vi "ObtainPrivateQueues.vi"(8 "error in (no error)":errorcluster, 11 "DAQmx":refnum<class "DAQmx.lvclass">) -> (0 "error out":errorcluster, 3 "DAQmx out":refnum<class "DAQmx.lvclass">)   [LabVIEW 2019, in "DAQmx.lvclass"]
uses:
  DAQmx.lvclass
  typedefs/DAQmx.States--enum.ctl
  typedefs/DAQ.Config.AO--Cluster--Array.ctl
  typedefs/DAQ.Config.AO--Cluster.ctl
  typedefs/DAQ.Config.AO.Range--enum.ctl
  typedefs/DAQ.Config.Device Type--enum.ctl
  typedefs/DAQ.Config.AI--Cluster--Array.ctl
  typedefs/DAQ.Config.AI--Cluster.ctl
  typedefs/DAQ.Config.AI.Coupling--enum.ctl
  typedefs/DAQ.Config.AI.Range--enum.ctl
  typedefs/DAQ.Config.Timing--Cluster.ctl
  typedefs/DAQ.Config.Timing.Sampling--Cluster.ctl
  typedefs/DAQ.Config.Timing.Fs Mode--enum.ctl
  DAQmx.lvclass/DAQmx.ctl
panel:
  # "For instructions on how to use the JKI State Machine Objects, examples and video tutorials, visit:\nhttp://jki.net/state-machine-objects/\n\nJKI State Machine Objects™\nhttp://jki.net/state-machine-objects/\nCopyright (C) 2005-2015, JKI <info@jki.net>\nALL RIGHTS RESERVED"
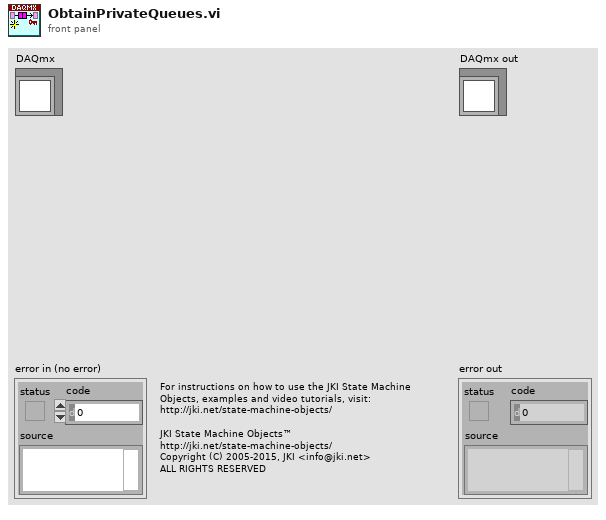
[diagram p1: front panel]
types:
  T1 = typedef "DAQmx.lvclass/DAQmx.States--enum.ctl" = enum16{"idle", "start", "stop", "calibrate", "auto", "exit"}
  T2 = typedef "DAQmx.lvclass/DAQ.Config.AO--Cluster--Array.ctl" = T3[]
  T3 = typedef "DAQmx.lvclass/DAQ.Config.AO--Cluster.ctl" = cluster{"Channels":tag, "Range":T4, "output terminal configuration":i32, "Type":T5}
  T4 = typedef "DAQmx.lvclass/DAQ.Config.AO.Range--enum.ctl" = enum16{"±0.1", "±1.0", "±10.0", ""}
  T5 = typedef "DAQmx.lvclass/DAQ.Config.Device Type--enum.ctl" = enum16{"None", "USB-4431", "PXI-446x"}
  T6 = typedef "DAQmx.lvclass/DAQ.Config.AI--Cluster--Array.ctl" = T7[]
  T7 = typedef "DAQmx.lvclass/DAQ.Config.AI--Cluster.ctl" = cluster{"Channels":tag, "Coupling":T8, "Range":T9, "input terminal configuration":i32, "Type":T5}
  T8 = typedef "DAQmx.lvclass/DAQ.Config.AI.Coupling--enum.ctl" = u16
  T9 = typedef "DAQmx.lvclass/DAQ.Config.AI.Range--enum.ctl" = enum16{"±0.316", "±1.00", "±3.16", "±10.0", "±31.6", "±42.4", ""}
  T10 = typedef "DAQmx.lvclass/DAQ.Config.Timing--Cluster.ctl" = cluster{"Sampling":T11, "sample mode":i32, "FsMode":T12, "Fs Multiplier":dbl, "Refresh Rate (Hz)":dbl, "Decimation.PreDSP":i32, "Decimation.PostDSP":i32, "Fs.Output":dbl}
  T11 = typedef "DAQmx.lvclass/DAQ.Config.Timing.Sampling--Cluster.ctl" = cluster{"Fs":dbl, "#s":i32}
  T12 = typedef "DAQmx.lvclass/DAQ.Config.Timing.Fs Mode--enum.ctl" = enum16{"Manual", "Auto Fs", "Max Fs"}
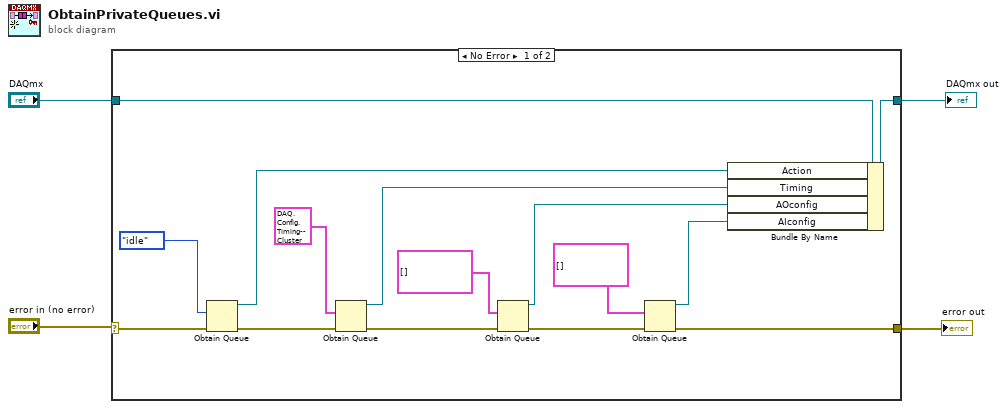
[diagram p0: block diagram]
diagram:
  n1 = case shown="No Error" "error in (no error)" {
    selector: "error in (no error)" -> [w16 w21]
    tunnel: [w8 w21] -> w2
    tunnel: [w18 w20] -> w3
    tunnel: "DAQmx" -> [w19 w20]
    frame No Error {
      n2 = Obtain Queue(element data type=DAQmx.States--enum."idle", error in (no error)=w16) -> (queue out=w9:refnum<queue>, error out=w15:errorcluster)  [unwired: 3 in, 1 out]
      n3 = Obtain Queue(element data type=T10 {"Sampling"={"Fs"=1000.0, "#s"=128}, "sample mode"=10123, "FsMode"=enum."Manual", "Fs Multiplier"=1.0, "Refresh Rate (Hz)"=10.0, "Decimation.PreDSP"=1, "Decimation.PostDSP"=1, "Fs.Output"=204789.0}, error in (no error)=w15) -> (queue out=w6:refnum<queue>, error out=w14:errorcluster)  [unwired: 3 in, 1 out]
      n4 = Obtain Queue(element data type=T2 [], error in (no error)=w14) -> (queue out=w5:refnum<queue>, error out=w13:errorcluster)  [unwired: 3 in, 1 out]
      n5 = Obtain Queue(element data type=T6 [], error in (no error)=w13) -> (queue out=w12:refnum<queue>, error out=w8:errorcluster)  [unwired: 3 in, 1 out]
      n6 = Bundle By Name(cluster=w19, "Action"=w9, "Timing"=w6, "AOconfig"=w5, "AIconfig"=w12) -> (w18:refnum<class "DAQmx.lvclass">)
    }
    frame Error {
    }
  }
  "error out" <- w2
  "DAQmx out" <- w3
